vi "Execute Command On Target.vi"(6 "wait for reply (T)":bool=TRUE, 8 "error in":errorcluster, 10 "Command":string, 11 "Module ID":i32=-1) -> (0 "error out":errorcluster, 1 "timed out?":bool, 2 "Errors":T1[](array[typedef]), 3 "Status":T2, 4 "Output":string, 5 "Sent Command":string)   [LabVIEW 2015, in "LV-WinSCP.lvlib"]
doc: "This request allows executing a command on the destination target.\nIt synchronously get the output and errors if any and publishes them in the reply and through a broadcast. If the command return time may overpass the module timeout, do not wait for reply and use the broadcast instead to get the output and errors.\n\nThe command <b>MUST NOT</b> be blocking ! Otherwise this VI will never stop executing.\nFor example, never use 'top' command with this method.\n\nTo use this VI, the target must expose a SSH shell.\n_____\nCreated using DQMH Event Scripter 6.1.0.128."
uses:
  LV-WinSCP.lvlib
  Classes/CommandExecution/Status.ctl
  Classes/CommandExecution/ErrorDescription.ctl
  Execute Command On Target Argument--cluster.ctl
  Execute Command On Target (Reply Payload)--cluster.ctl
  Classes/CommandExecution/Command Execution.lvclass
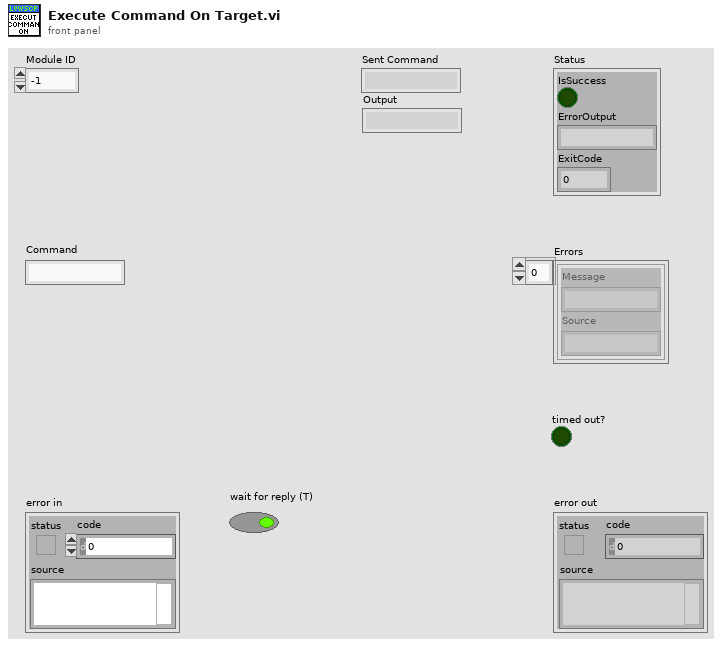
[diagram p1: front panel]
types:
  T1 = typedef "WinSCP.lvlib/Command Execution.lvclass/ErrorDescription.ctl" = cluster{"Message":string, "Source":string}
  T2 = typedef "WinSCP.lvlib/Command Execution.lvclass/Status.ctl" = cluster{"IsSuccess":bool, "ErrorOutput":string, "ExitCode":i32}
  T3 = typedef "LV-WinSCP.lvlib/Execute Command On Target Argument--cluster.ctl" = cluster{"Module ID":i32, "Command":string, "Wait Notifier":refnum<notifier>, "wait for reply":bool}
  T4 = typedef "LV-WinSCP.lvlib/Request Events--cluster.ctl" = cluster{"Stop Module":refnum<user-event>, "Show Panel":refnum<user-event>, "Hide Panel":refnum<user-event>, "Show Diagram":refnum<user-event>, "Get Module Execution Status":refnum<user-event>, "Initialize Session":refnum<user-event>, "Close Session":refnum<user-event>, "List Directory":refnum<user-event>, "Get Items From Target":refnum<user-event>, "Execute Command On Target":refnum<user-event>, "Send Items To Target":refnum<user-event>}
  T5 = typedef "LV-WinSCP.lvlib/Execute Command On Target (Reply Payload)--cluster.ctl" = cluster{"Status":T2, "Errors":T1[], "Sent Command":string, "error":errorcluster, "Output":string}
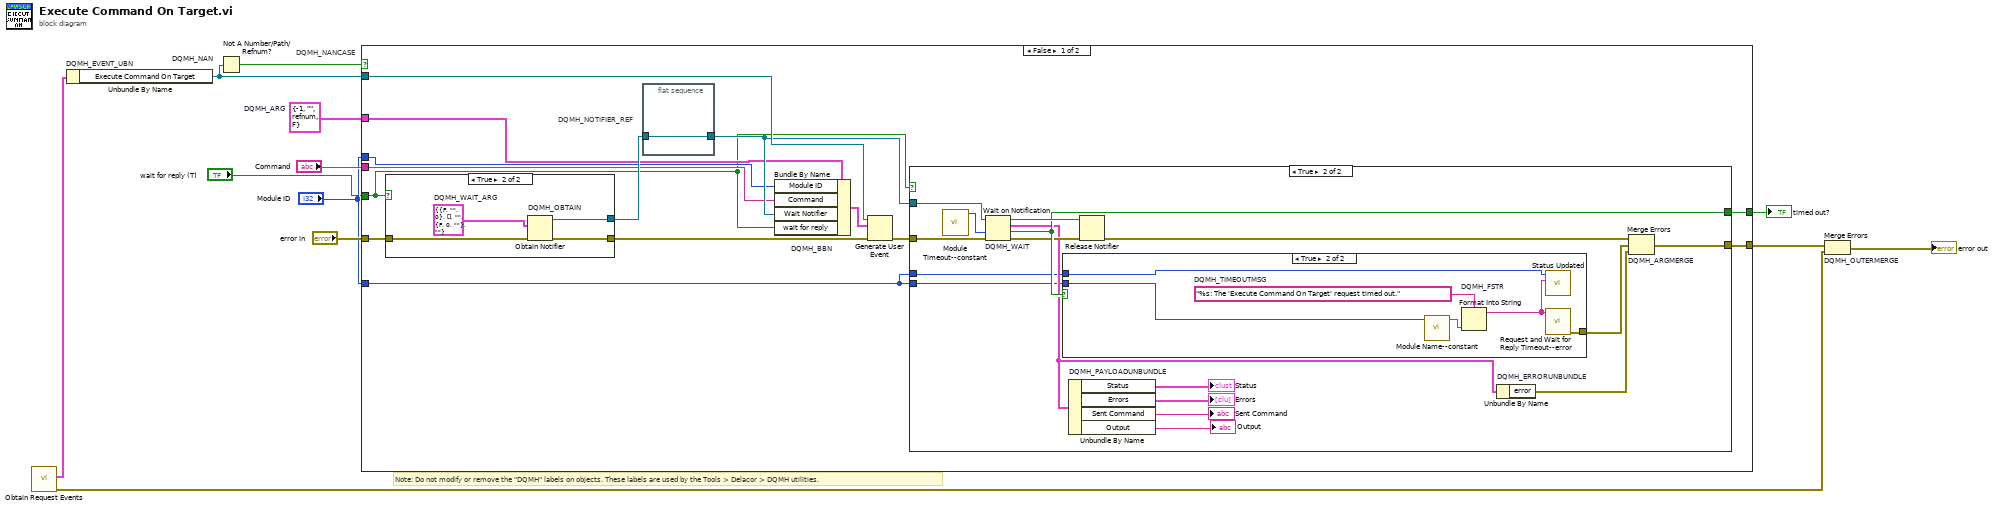
[diagram p0: block diagram]
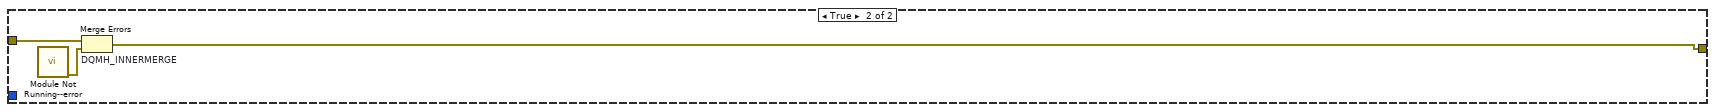
[diagram p5: hidden frame]
diagram:
  w6 = T3 {"Module ID"=-1, "Command"="", "Wait Notifier"=refnum, "wait for reply"=FALSE}  # DQMH_ARG
  # "Note: Do not modify or remove the \"DQMH\" labels on objects. These labels are used by the Tools > Delacor > DQMH utilities."
  n1 = call "Obtain Request Events.vi"() -> ("error out"=w2:errorcluster, "LV-WinSCP Request Events"=w1:T4)  [unwired: 10 in]
  n2 = Unbundle By Name "DQMH_EVENT_UBN"(w1) -> ("Execute Command On Target"=w10:refnum<user-event>)
  n3 = Not A Number/Path/Refnum? "DQMH_NAN"(number/path/refnum=w10) -> (NaN/Path/Refnum?=w9:bool)
  n4 = case "DQMH_NANCASE" shown="False" w9 {
    tunnel: "error in" -> [w26 w59]
    tunnel: w10 -> [w24 _]
    tunnel: [w21 w58] -> w7
    tunnel: [w22 _] -> w8
    tunnel: w6 -> [w17 _]
    tunnel: "Module ID" -> [w16 _]
    tunnel: "Command" -> [w15 _]
    tunnel: "Module ID" -> [w14 _]
    tunnel: "wait for reply (T)" -> [w13 _]
    frame False {
      n5 = case shown="True" w13 {
        tunnel: w26 -> [w52 w56]
        tunnel: [w52 w55] -> w23
        tunnel: [_ w53] -> w19
        frame False {
        }
        frame True {
          w54 = T5 {"Status"={"IsSuccess"=FALSE, "ErrorOutput"="", "ExitCode"=0}, "Errors"=[], "Sent Command"="", "error"={"status"=FALSE, "code"=0, "source"=""}, "Output"=""}  # DQMH_WAIT_ARG
          n6 = Obtain Notifier "DQMH_OBTAIN"(notification data type=w54, error in (no error)=w56) -> (notifier out=w53:refnum<notifier>, error out=w55:errorcluster)  [unwired: 2 in, 1 out]
        }
      }
      n7 = flat-sequence "DQMH_NOTIFIER_REF" {
        tunnel: w19 -> [w27]
        tunnel: [w27] -> w18
        frame #0 {
        }
      }
      n8 = Bundle By Name "DQMH_BBN"(cluster=w17, "Module ID"=w16, "Command"=w15, "Wait Notifier"=w18, "wait for reply"=w13) -> (w20:T3)
      n9 = Generate User Event(user event=w24, event data cluster=w20, error in=w23) -> (error out=w25:errorcluster)  [unwired: 1 in, 1 out]
      n10 = case shown="True" w13 {
        tunnel: w25 -> [w28 w45]
        tunnel: w18 -> [_ w44]
        tunnel: [_ w42] -> w22
        tunnel: [w28 w41] -> w21
        tunnel: w14 -> [_ w31]
        tunnel: w14 -> [_ w30]
        frame False {
        }
        frame True {
          n11 = call "Module Timeout--constant.vi"() -> ("Module Timeout"=w35:i32)  [unwired: 11 in]
          n12 = Wait on Notification "DQMH_WAIT"(notifier=w44, timeout in ms (-1)=w35, error in (no error)=w45) -> (notifier out=w43:refnum<notifier>, notification=w36:T5, timed out?=w42:bool, error out=w40:errorcluster)  [unwired: 1 in]
          n13 = case shown="True" w42 {
            tunnel: [_ w49] -> w37
            tunnel: w31 -> [_ w47]
            tunnel: w30 -> [_ w46]
            frame False {
            }
            frame True {
              w51 = "%s: The 'Execute Command On Target' request timed out."  # DQMH_TIMEOUTMSG
              n14 = call "Module Name--constant.vi"("Module ID"=w46) -> ("Module Name"=w48:string)  [unwired: 10 in]
              n15 = Format Into String "DQMH_FSTR"(format string=w51, w48) -> (resulting string=w50:string)  [unwired: 2 in, 1 out]
              n16 = call "Status Updated.vi"("Status"=w50, "Module ID"=w47) -> ()  [unwired: 9 in, 1 out]
              n17 = call "Request and Wait for Reply Timeout--error.vi"("Error Message"=w50) -> ("error out"=w49:errorcluster)  [unwired: 10 in]
            }
          }
          n18 = Unbundle By Name "DQMH_PAYLOADUNBUNDLE"(w36) -> ("Status"=→"Status":T2, "Errors"=→"Errors":T1[], "Sent Command"=→"Sent Command":string, "Output"=→"Output":string)
          n19 = Release Notifier(notifier=w43, error in (no error)=w40) -> (error out=w39:errorcluster)  [unwired: 1 in, 2 out]
          n20 = Unbundle By Name "DQMH_ERRORUNBUNDLE"(w36) -> ("error"=w38:errorcluster)
          n21 = Merge Errors "DQMH_ARGMERGE"(w39, w37, w38) -> (w41:errorcluster)
        }
      }
    }
    frame True {
      n22 = call "Module Not Running--error.vi"() -> ("error out"=w57:errorcluster)  [unwired: 11 in]
      n23 = Merge Errors "DQMH_INNERMERGE"(w59, w57) -> (w58:errorcluster)
    }
  }
  "timed out?" <- w8
  n24 = Merge Errors "DQMH_OUTERMERGE"(w7, w2) -> (→"error out":errorcluster)
